vi "GetLimsTestStep.vi"(8 "error in (no error)":errorcluster, 10 "step-id":i32, 11 "ByteGSAPIBase in":refnum<class "ByteQXAPIBase.lvclass">) -> (0 "error out":errorcluster, 2 "StepList":T1, 3 "ByteGSAPIBase out":refnum<class "ByteQXAPIBase.lvclass">)   [LabVIEW 2019, in "ByteQXWebAPI.lvlib" / "ByteQXAPIBase.lvclass"]
doc: "Obtain a single step based on the step-id"
uses:
  ByteQXAPIBase.lvclass
  TypeDef/Step.ctl
  TypeDef/Asset.ctl
  Private/module.ctl
  ByteQXAPIBase.lvclass/ByteQXAPIBase.ctl
  <vilib>/Bytelabs/ByteREST/ByteRESTClass/ByteRESTBase/RESTBase.lvclass
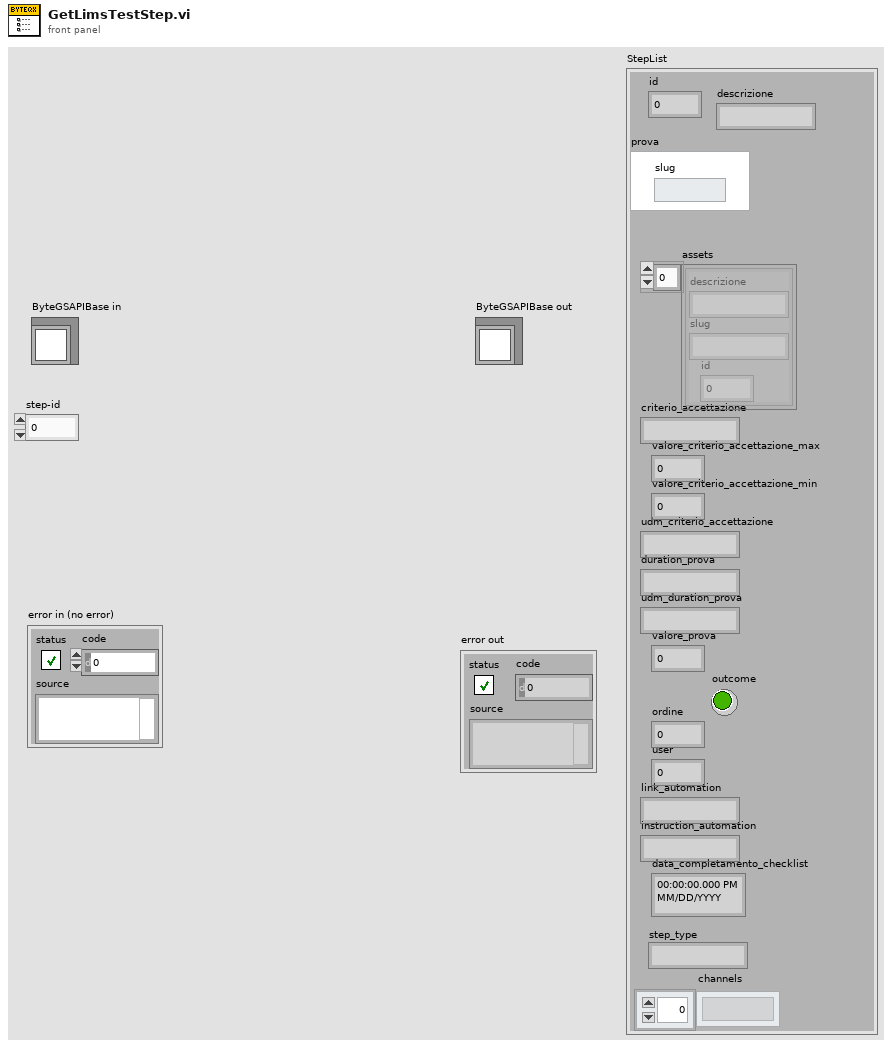
[diagram p1: front panel]
types:
  T1 = typedef "ByteQXWebAPI.lvlib/ByteQXAPIBase.lvclass/Step.ctl" = cluster{"id":i32, "descrizione":string, "prova":cluster{"slug":string}, "assets":T2[], "criterio_accettazione":string, "valore_criterio_accettazione_max":dbl, "valore_criterio_accettazione_min":dbl, "udm_criterio_accettazione":string, "duration_prova":string, "udm_duration_prova":string, "valore_prova":dbl, "ordine":i32, "user":i32, "link_automation":string, "instruction_automation":string, "data_completamento_checklist":timestamp, "outcome":bool, "step_type":string, "channels":string[]}
  T2 = typedef "ByteQXWebAPI.lvlib/ByteQXAPIBase.lvclass/Asset.ctl" = cluster{"descrizione":string, "slug":string, "id":i32}
  T3 = typedef "ByteQXWebAPI.lvlib/ByteQXAPIBase.lvclass/module.ctl" = enum16{"gs", "tms"}
  T4 = cluster{"id":i32, "descrizione":string, "assets":T2[], "criterio_accettazione":string, "valore_criterio_accettazione_max":dbl, "valore_criterio_accettazione_min":dbl, "udm_criterio_accettazione":string, "duration_prova":string, "udm_duration_prova":string, "data_completamento_checklist":string, "valore_prova":dbl, "outcome":string, "ordine":i32, "user":i32, "link_automation":string, "instruction_automation":string, "channels":string[], "step_type":string, "prova":cluster{"slug":string}}[]
  T5 = cluster{"id":i32, "descrizione":string, "assets":T2[], "criterio_accettazione":string, "valore_criterio_accettazione_max":dbl, "valore_criterio_accettazione_min":dbl, "udm_criterio_accettazione":string, "duration_prova":string, "udm_duration_prova":string, "data_completamento_checklist":string, "valore_prova":dbl, "outcome":string, "ordine":i32, "user":i32, "link_automation":string, "instruction_automation":string, "channels":string[], "step_type":string, "prova":cluster{"slug":string}}
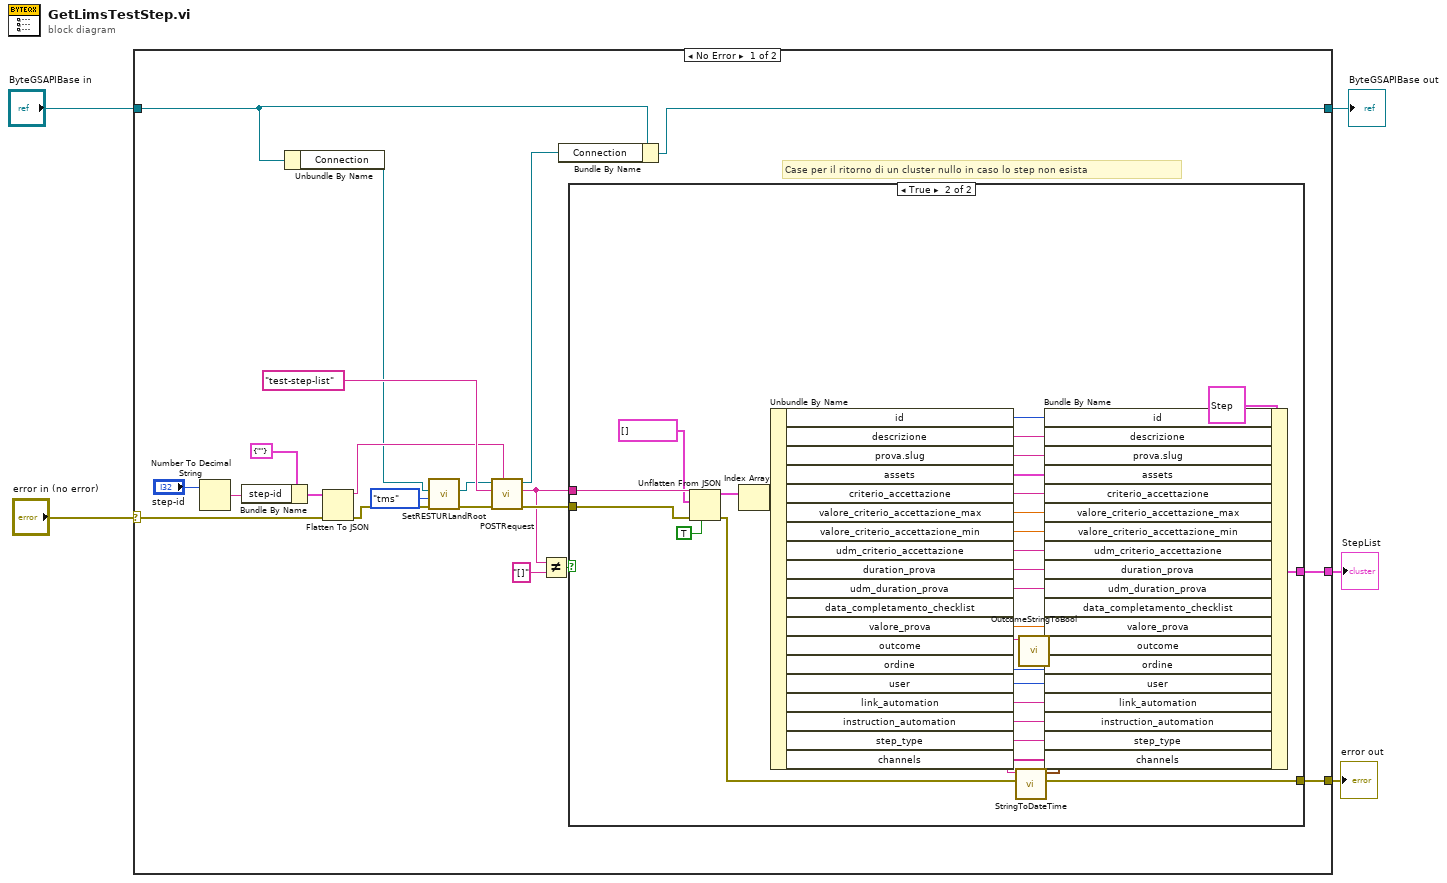
[diagram p0: block diagram]
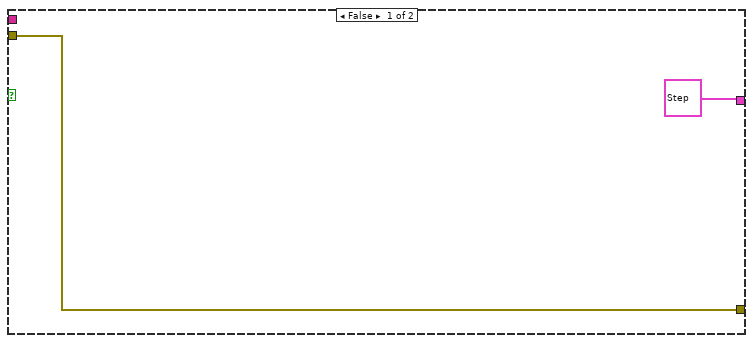
[diagram p2: hidden frame]
diagram:
  n1 = case shown="No Error" "error in (no error)" {
    selector: "error in (no error)" -> [w17 w61]
    tunnel: [w15 w61] -> w4
    tunnel: [w24 w60] -> w2
    tunnel: "ByteGSAPIBase in" -> [w25 w60]
    tunnel: [w14 _] -> w1
    frame No Error {
      # "Case per il ritorno di un cluster nullo in caso lo step non esista"
      n2 = Number To Decimal String(number="step-id") -> (decimal integer string=w21:string)  [unwired: 1 in]
      n3 = Bundle By Name(cluster=cluster{"step-id":string} {"step-id"=""} ("Request"), "step-id"=w21) -> (w19:cluster{"step-id":string})
      n4 = Unbundle By Name(w25) -> ("Connection"=w8:refnum<class "RESTBase.lvclass">)
      n5 = Flatten To JSON(anything=w19, error in (no error)=w17) -> (JSON string=w18:string, 11:w10:errorcluster)  [unwired: 1 in]
      n6 = call "SetRESTURLandRoot.vi"("error in (no error)"=w10, "module"=module."tms", "ByteREST in"=w8) -> ("error out"=w9:errorcluster, "ByteREST out"=w7:refnum<class "RESTBase.lvclass">)  [unwired: 7 in]
      n7 = call-dynamic "POSTRequest.vi"("Body in"=w18, "error in (no error)"=w9, "Request"="test-step-list", "ByteRESTBase in"=w7) -> ("error out"=w16:errorcluster, "Body"=w12:string, "ByteRESTBase out"=w26:refnum<class "RESTBase.lvclass">)  [unwired: 4 in, 1 out]
      n8 = Not Equal?(x=w12, y="[]") -> (x != y?=w13:bool)
      n9 = Bundle By Name(cluster=w25, "Connection"=w26) -> (w24:refnum<class "ByteQXAPIBase.lvclass">)
      n10 = case shown="True" w13 {
        tunnel: w12 -> [_ w59]
        tunnel: w16 -> [w28 w58]
        tunnel: [w28 w40] -> w15
        tunnel: [T1 {"id"=0, "descrizione"="", "prova"={"slug"=""}, "assets"=[], "criterio_accettazione"="", "valore_criterio_accettazione_max"=0.0, "valore_criterio_accettazione_min"=0.0, "udm_criterio_accettazione"="", "duration_prova"="", "udm_duration_prova"="", "valore_prova"=0.0, "ordine"=0, "user"=0, "link_automation"="", "instruction_automation"="", "data_completamento_checklist"=timestamp(0 s since 1904-01-01), "outcome"=FALSE, "step_type"="", "channels"=[]} ("StepList") w37] -> w14
        frame False {
        }
        frame True {
          n11 = Unflatten From JSON(JSON string=w59, type and defaults=T4 [], default null elements? (F)=TRUE, error in (no error)=w58) -> (value=w34:T4, error out=w39:errorcluster)  [unwired: 3 in]
          n12 = Index Array(array=w34) -> (element=w35:T5)  [unwired: 1 in]
          n13 = Unbundle By Name(w35) -> ("id"=w41:i32, "descrizione"=w42:string, "prova.slug"=w43:string, "assets"=w44:T2[], "criterio_accettazione"=w45:string, "valore_criterio_accettazione_max"=w46:dbl, "valore_criterio_accettazione_min"=w47:dbl, "udm_criterio_accettazione"=w48:string, "duration_prova"=w49:string, "udm_duration_prova"=w50:string, "data_completamento_checklist"=w51:string, "valore_prova"=w53:dbl, "outcome"=w32:string, "ordine"=w54:i32, "user"=w55:i32, "link_automation"=w56:string, "instruction_automation"=w57:string, "step_type"=w30:string, "channels"=w29:string[])
          n14 = call "StringToDateTime.vi"("error in (no error)"=w39, "datetime string"=w51) -> ("error out"=w40:errorcluster, "timestamp"=w52:timestamp)  [unwired: 8 in]
          n15 = call "OutcomeStringToBool.vi"("outcome string"=w32) -> ("outcome bool"=w31:bool)  [unwired: 10 in]
          n16 = Bundle By Name(cluster=T1 {"id"=0, "descrizione"="", "prova"={"slug"=""}, "assets"=[], "criterio_accettazione"="", "valore_criterio_accettazione_max"=0.0, "valore_criterio_accettazione_min"=0.0, "udm_criterio_accettazione"="", "duration_prova"="", "udm_duration_prova"="", "valore_prova"=0.0, "ordine"=0, "user"=0, "link_automation"="", "instruction_automation"="", "data_completamento_checklist"=timestamp(0 s since 1904-01-01), "outcome"=FALSE, "step_type"="", "channels"=[]} ("StepList"), "id"=w41, "descrizione"=w42, "prova.slug"=w43, "assets"=w44, "criterio_accettazione"=w45, "valore_criterio_accettazione_max"=w46, "valore_criterio_accettazione_min"=w47, "udm_criterio_accettazione"=w48, "duration_prova"=w49, "udm_duration_prova"=w50, "data_completamento_checklist"=w52, "valore_prova"=w53, "outcome"=w31, "ordine"=w54, "user"=w55, "link_automation"=w56, "instruction_automation"=w57, "step_type"=w30, "channels"=w29) -> (w37:T1)
        }
      }
    }
    frame Error {
    }
  }
  "error out" <- w4
  "ByteGSAPIBase out" <- w2
  "StepList" <- w1
